vi "receiveTEDS.vi"(8 "error in (no error)":errorcluster, 11 "ILC in":refnum<class "ILC.lvclass">) -> (0 "error out":errorcluster, 2 "TEDS Memory":T1, 3 "ILC out":refnum<class "ILC.lvclass">)   [LabVIEW 2015, in "ILCCommon.lvlib" / "ILC.lvclass"]
uses:
  <userlib>/Common/ILC/ILC/ILC.lvclass
  <userlib>/Common/ILC/Typedefs/TEDS.ctl
  <userlib>/Common/ILC/ILCModelTypedefs/FinalDelimiter.ctl
  <userlib>/Common/ILC/ILC/ILC.lvclass/ILC.ctl
  <userlib>/Common/ILC/ILCModelTypedefs/ILCModelTypedefs.lvlib
  <userlib>/Common/ILC/Typedefs/ILCTypedefs.lvlib
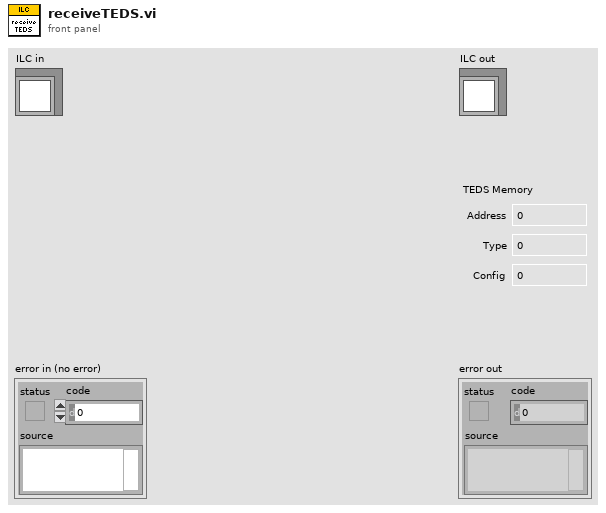
[diagram p1: front panel]
types:
  T1 = typedef "ILCCommon.lvlib/ILCTypedefs.lvlib/TEDS.ctl" = cluster{"Address":i32, "Type":i32, "Config":i32}
  T2 = typedef "ILCCommon.lvlib/ILCModelTypedefs.lvlib/FinalDelimiter.ctl" = enum16{",", "<CR><LF>"}
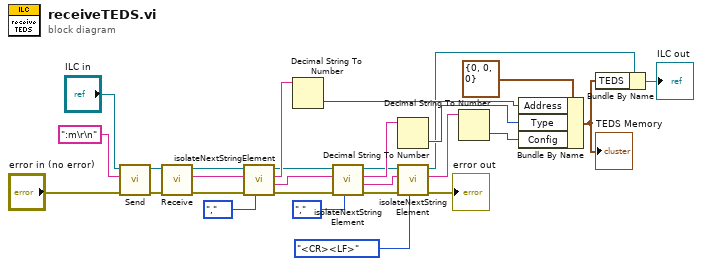
[diagram p0: block diagram]
diagram:
  n1 = call-dynamic "Send.vi"("error in (no error)"="error in (no error)", "Message"=":m\r\n", "ILC in"="ILC in") -> ("error out"=w3:errorcluster, "ILC out"=w7:refnum<class "ILC.lvclass">)  [unwired: 7 in]
  n2 = call-dynamic "Receive.vi"("error in (no error)"=w3, "ILC in"=w7) -> ("error out"=w4:errorcluster, "Response"=w5:string, "ILC out"=w6:refnum<class "ILC.lvclass">)  [unwired: 7 in]
  n3 = call <userlib>:"isolateNextStringElement.vi"("Final Delimiter"=FinalDelimiter.",", "error in (no error)"=w4, "inputString"=w5, "ILC in"=w6) -> ("error out"=w14:errorcluster, "remainingString"=w19:string, "extractedSegment"=w20:string, "ILC out"=w18:refnum<class "ILC.lvclass">)  [unwired: 4 in]
  n4 = Decimal String To Number(string=w20) -> (number=w25:i32)  [unwired: 2 in, 1 out]
  n5 = call <userlib>:"isolateNextStringElement.vi"("Final Delimiter"=FinalDelimiter.",", "error in (no error)"=w14, "inputString"=w19, "ILC in"=w18) -> ("error out"=w13:errorcluster, "remainingString"=w22:string, "extractedSegment"=w23:string, "ILC out"=w21:refnum<class "ILC.lvclass">)  [unwired: 4 in]
  n6 = Decimal String To Number(string=w23) -> (number=w26:i32)  [unwired: 2 in, 1 out]
  n7 = call <userlib>:"isolateNextStringElement.vi"("Final Delimiter"=FinalDelimiter."<CR><LF>", "error in (no error)"=w13, "inputString"=w22, "ILC in"=w21) -> ("error out"=→"error out":errorcluster, "extractedSegment"=w24:string, "ILC out"=w12:refnum<class "ILC.lvclass">)  [unwired: 4 in, 1 out]
  n8 = Decimal String To Number(string=w24) -> (number=w27:i32)  [unwired: 2 in, 1 out]
  n9 = Bundle By Name(cluster=T1 {"Address"=0, "Type"=0, "Config"=0} ("TEDS Memory"), "Address"=w25, "Type"=w26, "Config"=w27) -> (w16:T1)
  "TEDS Memory" <- w16
  n10 = Bundle By Name(cluster=w12, "TEDS"=w16) -> (→"ILC out":refnum<class "ILC.lvclass">)
